vi "Read Slave ID.vi"(8 "error in (no error)":errorcluster, 11 "MB PLC in":refnum<class "MB PLC Client.lvclass">) -> (0 "error out":errorcluster, 2 "Slave ID":u8=1, 3 "MB PLC out":refnum<class "MB PLC Client.lvclass">)   [LabVIEW 2018, in "MB PLC Client.lvlib" / "MB PLC Client.lvclass"]
uses:
  MB PLC Client.lvclass
  MB PLC Client.lvclass/MB PLC Client.ctl
  <vilib>/Plasmionique/MB Master/MB_Master/MB_Master.lvclass
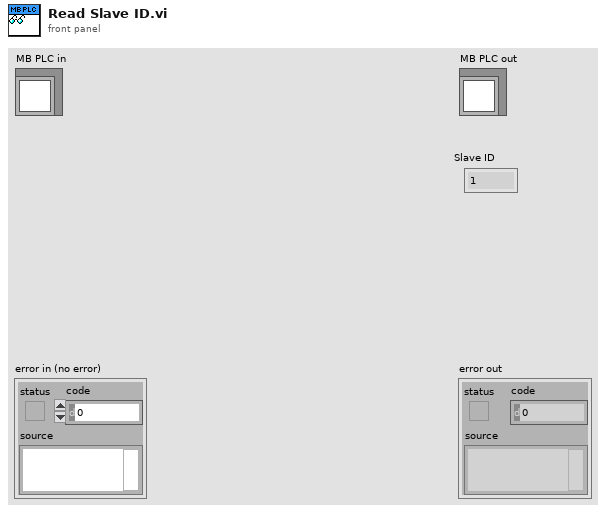
[diagram p1: front panel]
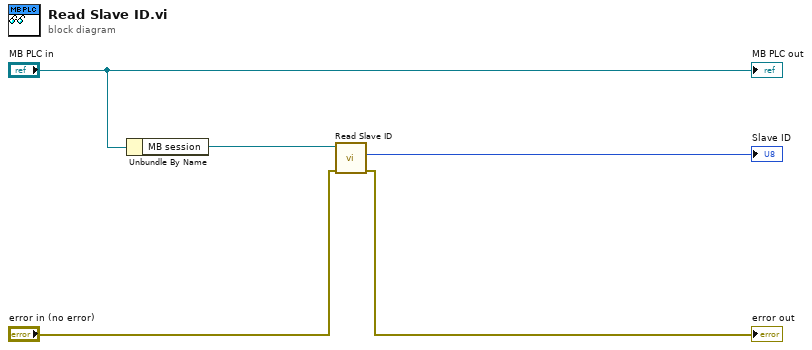
[diagram p0: block diagram]
diagram:
  n1 = Unbundle By Name("MB PLC in") -> ("MB session"=w4:refnum<class "MB_Master.lvclass">)
  n2 = call-dynamic "Read Slave ID.vi"("error in (no error)"="error in (no error)", "MB_Master in"=w4) -> ("error out"=→"error out":errorcluster, "Slave ID"=→"Slave ID":u8)  [unwired: 7 in, 1 out]
  "MB PLC out" <- "MB PLC in"
